vi "ArraySerpentineToImage.vi"(0 "DataIn":dbl[](array[numeric]), 1 "N":i32) -> (2 "DataOut":dbl[][](array[numeric]))   [LabVIEW 2009]
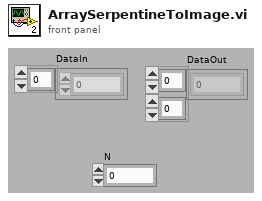
[diagram p1: front panel]
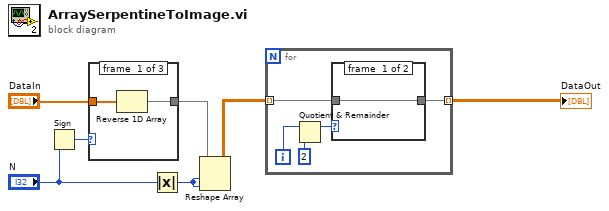
[diagram p0: block diagram]
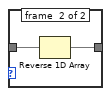
[diagram p4: hidden frame]
diagram:
  n1 = Sign(1:"N") -> (0:w3:i32)
  n2 = case shown="0, Default" w3 {
    tunnel: "DataIn" -> [w9 w10 w11]
    tunnel: [w8 w10 w11] -> w1
    frame #0 {
      n3 = Reverse 1D Array(array=w9) -> (reversed array=w8:dbl[])
    }
    frame #1 {
    }
    frame #2 {
    }
  }
  n4 = Absolute Value(x="N") -> (abs(x)=w5:i32)
  n5 = Reshape Array(w1, w5, w5) -> (w7:dbl[][])
  n6 = for {
    tunnel: w7 -> [w15] mode=indexing
    tunnel: [w14] -> w6 mode=indexing
    i -> [w13]
    n7 = Quotient & Remainder(x=w13, y=2) -> (x-y*floor(x/y)=w12:i32)  [unwired: 1 out]
    n8 = case shown="0, Default" w12 {
      tunnel: w15 -> [w17 w19]
      tunnel: [w17 w18] -> w14
      frame #0 {
      }
      frame #1 {
        n9 = Reverse 1D Array(array=w19) -> (reversed array=w18:dbl[])
      }
    }
  }
  "DataOut" <- w6
